vi "array_to_memo_admin.vi"(11 "memory":u8[](array[numeric])) -> (3 "?":T1)   [LabVIEW 2015, in "PolyVIEW.lvclass"]
uses:
  PolyVIEW.lvclass
  Admin memo.ctl
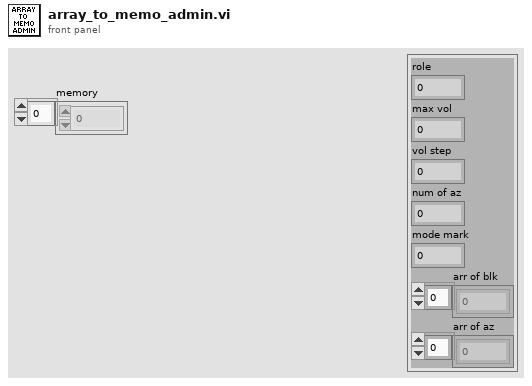
[diagram p1: front panel]
types:
  T1 = typedef "Admin memo.ctl" = cluster{"role":i32, "max vol":i32, "vol step":i32, "num of az":i32, "mode mark":i32, "arr of blk":i32[], "arr of az":i32[]}
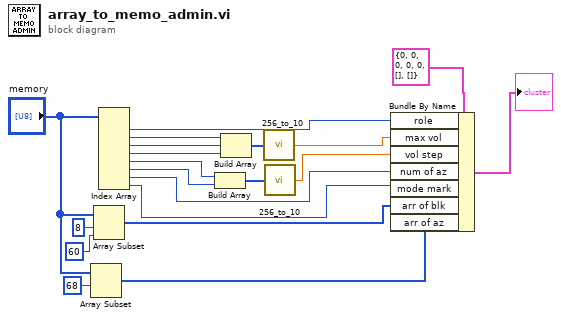
[diagram p0: block diagram]
diagram:
  n1 = Array Subset(array="memory", index=68) -> (w2:u8[])  [unwired: 1 in]
  n2 = Array Subset(array="memory", index=8, length=60) -> (w5:u8[])
  n3 = Index Array(array="memory") -> (element #1=w20:u8, element #2=w16:u8, element #3=w15:u8, element #4=w14:u8, element #5=w12:u8, element #6=w11:u8, element #7=w9:u8, element #8=w8:u8)  [unwired: 8 in]
  n4 = Build Array(w12, w11) -> (w18:u8[])
  n5 = Build Array(w16, w15, w14) -> (w19:u8[])
  n6 = call "256_to_10.vi"("Array"=w19) -> ("Numeric"=w13:dbl)
  n7 = call "256_to_10.vi"("Array"=w18) -> ("Numeric"=w10:dbl)
  n8 = Bundle By Name(cluster=T1 {"role"=0, "max vol"=0, "vol step"=0, "num of az"=0, "mode mark"=0, "arr of blk"=[], "arr of az"=[]}, "role"=w20, "max vol"=w13, "vol step"=w10, "num of az"=w9, "mode mark"=w8, "arr of blk"=w5, "arr of az"=w2) -> (→"?":T1)
